vi "MCL Monitor N.vi"(9 "handle":i32, 10 "axis":u32, 11 "position":dbl) -> (3 "function return":dbl)   [LabVIEW 2017, in "Madlib.lvlib"]
doc: "MADLIB_API double MCL_MonitorN(double position, unsigned int axis, int handle);"
uses:
  Madlib.lvlib
  Madlib.dll
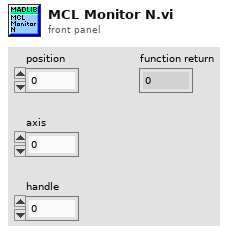
[diagram p1: front panel]
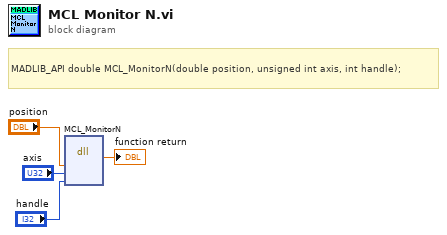
[diagram p0: block diagram]
diagram:
  # "MADLIB_API\tdouble\tMCL_MonitorN(double position, unsigned int axis, int handle);"
  n1 = dll-call lib="C:/Users/francesco/dev/pump-probe/Piezo/lvlib/Madlib.*" fn="MCL_MonitorN"("position"="position", "axis"="axis", "handle"="handle") -> (→"function return":dbl)  [unwired: 6 in, 2 out]
